vi "CmdDevice.vi"(8 "error in (no error)":errorcluster, 10 "Command:":string, 11 "reference in":refnum<k7>) -> (0 "error out":errorcluster, 2 "Response:":string, 3 "reference out":refnum<k7>)   [LabVIEW 2020]
panel:
  in  "DL_prog":string
  in  "Download PRG?":bool
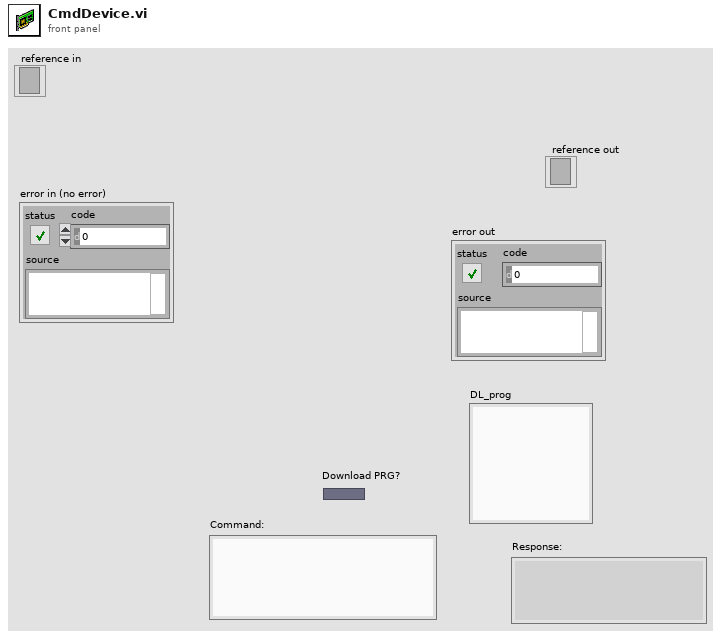
[diagram p1: front panel]
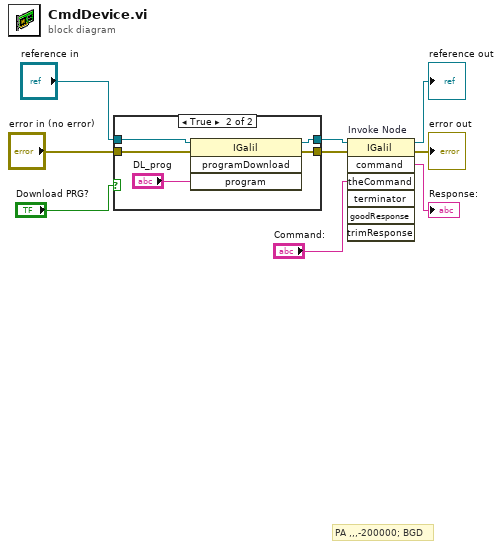
[diagram p0: block diagram]
diagram:
  # "PA ,,,-200000; BGD"
  n1 = case shown="True" "Download PRG?" {
    tunnel: [w10 w15] -> w9
    tunnel: "reference in" -> [w11 w14]
    tunnel: [w11 w13] -> w4
    tunnel: "error in (no error)" -> [w10 w12]
    frame False {
    }
    frame True {
      n2 = invoke class="IGalil" method="programDownload"(reference=w14, error in=w12, "program"="DL_prog") -> (reference out=w13:refnum<k7>, error out=w15:errorcluster)  [unwired: 1 in, 2 out]
    }
  }
  n3 = invoke on="Invoke Node" class="IGalil" method="command"(reference=w4, error in=w9, "theCommand"="Command:") -> (reference out=→"reference out":refnum<k7>, error out=→"error out":errorcluster, "command"=→"Response:":string)  [unwired: 4 in, 4 out]
